vi "Generate Page.vi"(8 "error in (no error)":errorcluster, 11 "Node Ptr":T1 format="%.0x") -> (0 "error out":errorcluster)   [LabVIEW 2013, in "Protection and Rolling Counter Addon System Explorer.lvlib"]
uses:
  Protection and Rolling Counter Addon System Explorer.lvlib
  <vilib>/NI Veristand/Custom Device API/Custom Device Item Ref.ctl
  <vilib>/NI Veristand/Custom Device API/Custom Device API.lvlib
panel:
  out "Frames":i32(listbox)
  in  "SHDocVw.IWebBrowser":refnum<k7>(container)
  in  "Header":cluster{"Section Name":string}={"Section Name"="Custom Device Item Settings"}
  in  "Description":string
  in  "Name":string
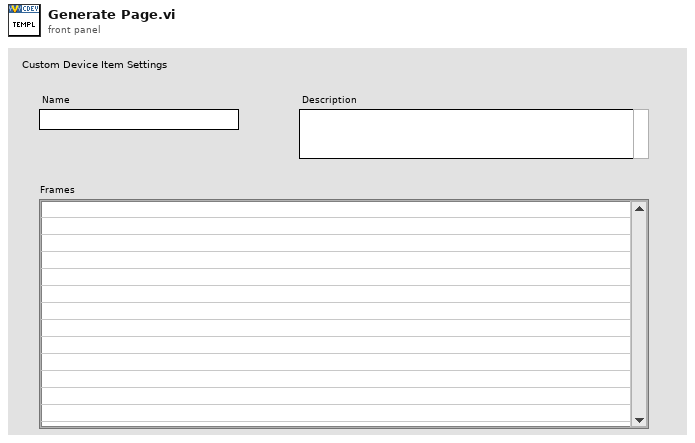
[diagram p1: front panel]
types:
  T1 = typedef "Custom Device API.lvlib/Custom Device Item Ref.ctl" = u64
  T2 = typedef "Custom Device API.lvlib/Custom Device Item Info.ctl" = cluster{"Name":string, "Is Channel":bool, "GUID":string, "Is Waveform":bool}
  T3 = typedef "Custom Device API.lvlib/Custom Device Commands.ctl" = enum16{"Default", "Item renamed", "Shutdown", "Dynamic button pressed"}
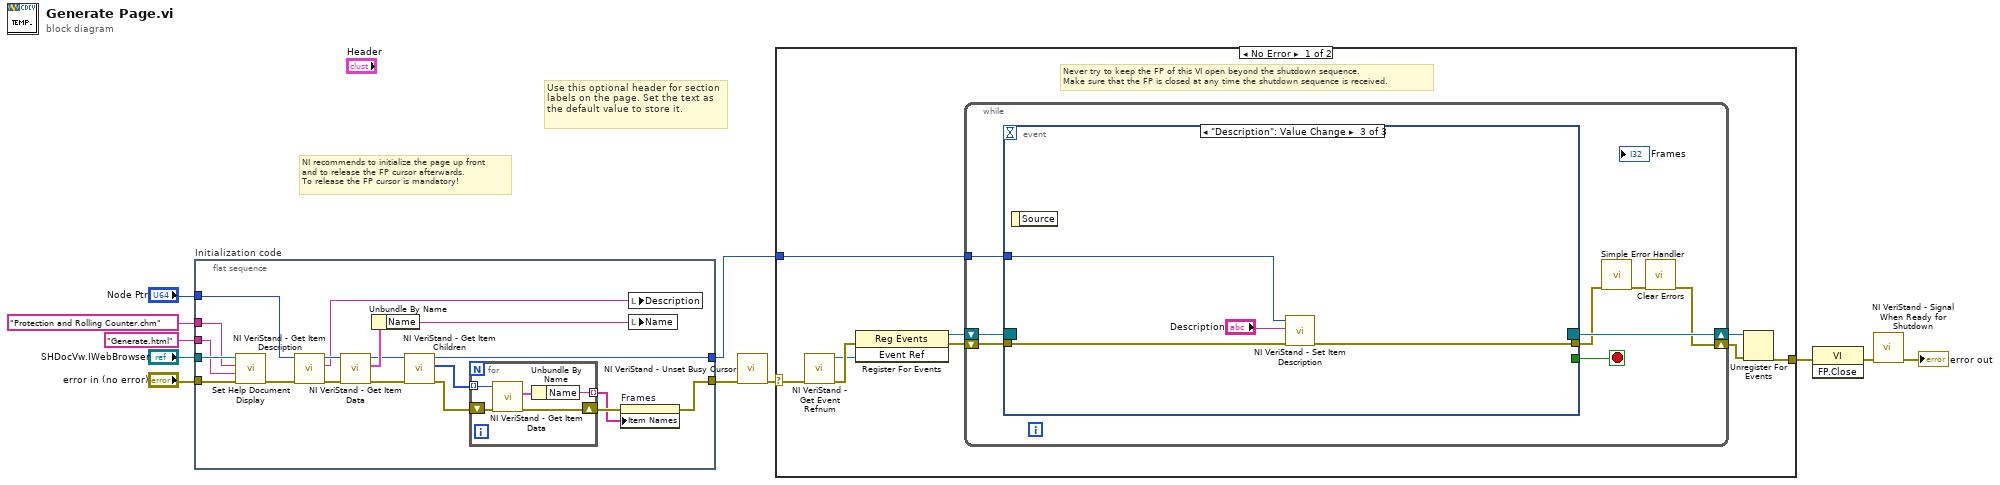
[diagram p0: block diagram]
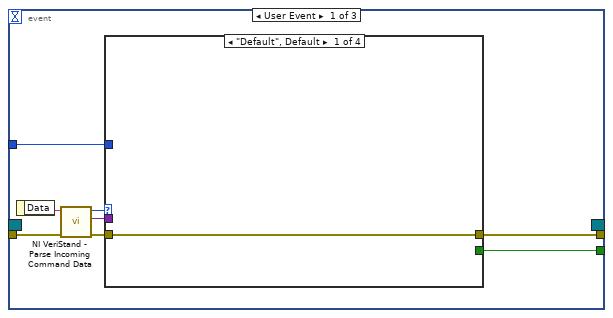
[diagram p2: hidden frame]
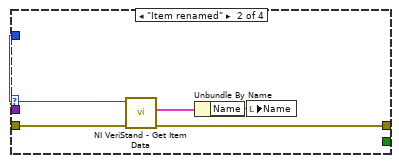
[diagram p3: hidden frame]
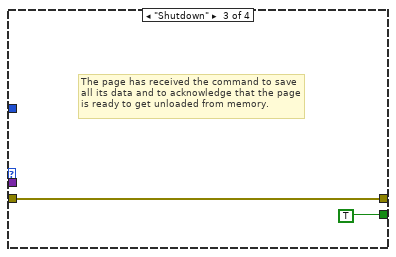
[diagram p4: hidden frame]
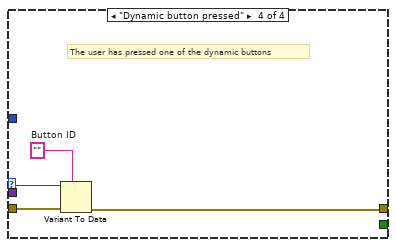
[diagram p5: hidden frame]
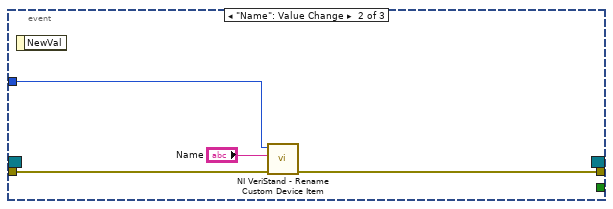
[diagram p6: hidden frame]
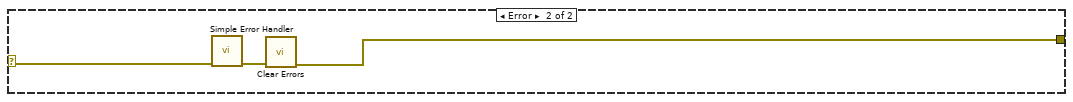
[diagram p7: hidden frame]
diagram:
  # "Use this optional header for section labels on the page. Set the text as the default value to store it."
  # "NI recommends to initialize the page up front\nand to release the FP cursor afterwards.\nTo release the FP cursor is mandatory!"
  n1 = flat-sequence "Initialization code" {
    tunnel: "error in (no error)" -> [w24]
    tunnel: "Node Ptr" -> [w29]
    tunnel: [w19] -> w7
    tunnel: [w16] -> w4
    tunnel: "SHDocVw.IWebBrowser" -> [w22]
    tunnel: "Generate.html" ("HTML File") -> [w21]
    tunnel: "Protection and Rolling Counter.chm" ("Main CHM File") -> [w20]
    frame #0 {
      n2 = call "Set Help Document Display.vi"("error in (no error)"=w24, "HTML File"=w21, "Main CHM File"=w20, "SHDocVw.IWebBrowser2"=w22) -> ("error out"=w23:errorcluster)  [unwired: 7 in]
      n3 = call <vilib>:"NI VeriStand - Get Item Description.vi"("error in (no error)"=w23, "Item Ref in"=w29) -> ("error out"=w27:errorcluster, "Description"=w28:string, "Item Ref out"=w30:T1)  [unwired: 7 out]
      n4 = call <vilib>:"NI VeriStand - Get Item Data.vi"("error in (no error)"=w27, "Item Ref in"=w30) -> ("error out"=w18:errorcluster, "Item Info"=w26:T2, "Item Ref out"=w17:T1)  [unwired: 7 out]
      n5 = Unbundle By Name(w26) -> ("Name"=w25:string)
      n6 = call <vilib>:"NI VeriStand - Get Item Children.vi"("error in (no error)"=w18, "Item Ref in"=w17) -> ("error out"=w15:errorcluster, "Child Refs"=w13:T1[], "Item Ref out"=w16:T1)  [unwired: 6 in, 1 out]
      n7 = for {
        shift-right: [w33] -> w14
        shift-left: w15 -> [w34]
        tunnel: w13 -> [w32] mode=indexing
        tunnel: [w31] -> w12 mode=indexing
        n8 = call <vilib>:"NI VeriStand - Get Item Data.vi"("error in (no error)"=w34, "Item Ref in"=w32) -> ("error out"=w33:errorcluster, "Item Info"=w35:T2)  [unwired: 8 out]
        n9 = Unbundle By Name(w35) -> ("Name"=w31:string)
      }
      n10 = property on="Frames" class="LstBox (strict)"(error in=w14, "Item Names"=w12) -> (error out=w19:errorcluster)  [unwired: 1 in, 1 out]
      n11 = local write "Description"(w28) -> ()
      n12 = local write "Name"(w25) -> ()
    }
  }
  n13 = call <vilib>:"NI VeriStand - Unset Busy Cursor.vi"("error in (no error)"=w7) -> ("error out"=w6:errorcluster)  [unwired: 10 out]
  n14 = case shown="No Error" w6 {
    selector: w6 -> [w36 w83]
    tunnel: [w41 w81] -> w11
    tunnel: w4 -> [w37 _]
    frame No Error {
      # "Never try to keep the FP of this VI open beyond the shutdown sequence.\nMake sure that the FP is closed at any time the shutdown sequence is received."
      n15 = call <vilib>:"NI VeriStand - Get Event Refnum.vi"("error in (no error)"=w36) -> ("error out"=w44:errorcluster, "Event Ref"=w40:refnum<user-event>)  [unwired: 9 out]
      n16 = register-events(error in=w44, w40) -> (reference out=w38:refnum<event-registration>, error out=w39:errorcluster)  [unwired: 1 in]
      n17 = while {
        tunnel: w37 -> [w48]
        shift-right: [w45] -> w42
        shift-left: w39 -> [w51]
        shift-right: [w52] -> w43
        shift-left: w38 -> [w50]
        stop <- w49 stop-if-true
        n18 = event shown="[2] \"Description\": Value Change" {
          selector: w50 -> [_ _ _]
          dyn-events: [_ _ _] -> w52
          timeout: _ -> [_ _ _]
          tunnel: w51 -> [w60 w76 w79]
          tunnel: [w56 _ _] -> w49
          tunnel: [w55 w75 w78] -> w47
          tunnel: w48 -> [w54 w74 w80]
          event User Event {
            n19 = event-data() -> ("Data"=w59:string)  [unwired: 1 out]
            n20 = call <vilib>:"NI VeriStand - Parse Incoming Command Data.vi"("error in (no error)"=w60, "Incoming data"=w59) -> ("error out"=w58:errorcluster, "Outgoing data"=w53:variant, "Action"=w57:T3)  [unwired: 7 out]
            n21 = case shown="\"Default\", Default" w57 {
              tunnel: w58 -> [w61 w66 w67 w72]
              tunnel: [_ _ TRUE _] -> w56
              tunnel: [w61 w63 w67 w69] -> w55
              tunnel: w54 -> [_ w65 _ _]
              tunnel: w53 -> [_ _ _ w71]
              frame "Default", Default {
              }
              frame "Item renamed" {
                n22 = call <vilib>:"NI VeriStand - Get Item Data.vi"("error in (no error)"=w66, "Item Ref in"=w65) -> ("error out"=w63:errorcluster, "Item Info"=w64:T2)  [unwired: 8 out]
                n23 = Unbundle By Name(w64) -> ("Name"=w62:string)
                n24 = local write "Name"(w62) -> ()
              }
              frame "Shutdown" {
                # "The page has received the command to save all its data and to acknowledge that the page is ready to get unloaded from memory."
              }
              frame "Dynamic button pressed" {
                w70 = ""  # Button ID
                # "The user has pressed one of the dynamic buttons"
                n25 = Variant To Data(error in=w72, type=w70, Variant=w71) -> (error out=w69:errorcluster)  [unwired: 1 out]
              }
            }
          }
          event "Name": Value Change {
            n26 = event-data() -> ()  [unwired: 2 out]
            n27 = call <vilib>:"NI VeriStand - Rename Custom Device Item.vi"("error in (no error)"=w76, "New Name"="Name", "Item Ref in"=w74) -> ("error out"=w75:errorcluster)  [unwired: 1 in, 7 out]
          }
          event "Description": Value Change {
            n28 = event-data() -> ()  [unwired: 2 out]
            n29 = call <vilib>:"NI VeriStand - Set Item Description.vi"("error in (no error)"=w79, "Description"="Description", "Item Ref in"=w80) -> ("error out"=w78:errorcluster)  [unwired: 8 out]
          }
        }
        n30 = call <vilib>:"Simple Error Handler.vi"("error in (no error)"=w47) -> ("error out"=w46:errorcluster)  [unwired: 1 in, 7 out]
        n31 = call <vilib>:"Clear Errors.vi"("error in (no error)"=w46) -> ("error out"=w45:errorcluster)  [unwired: 6 out]
      }
      n32 = Unregister For Events(event registration refnum=w43, error in=w42) -> (error out=w41:errorcluster)
    }
    frame Error {
      n33 = call <vilib>:"Simple Error Handler.vi"("error in (no error)"=w83) -> ("error out"=w82:errorcluster)  [unwired: 1 in, 7 out]
      n34 = call <vilib>:"Clear Errors.vi"("error in (no error)"=w82) -> ("error out"=w81:errorcluster)  [unwired: 6 out]
    }
  }
  n35 = invoke class="VI" method="FP.Close"(error in=w11) -> (error out=w10:errorcluster)  [unwired: 2 in, 2 out]
  n36 = call <vilib>:"NI VeriStand - Signal When Ready for Shutdown.vi"("error in (no error)"=w10) -> ("error out"=→"error out":errorcluster)  [unwired: 10 out]
